vi "createILC.vi"() -> (3 "ILC":refnum<class "ILC.lvclass">)   [LabVIEW 2016]
uses:
  Common_ILC/ILC/ILC.lvclass
  Common_SerialProtocols/SerialCommunicator/SerialCommunicator.lvclass
  Common_SerialProtocols/SerialProtocolFactory/SerialProtocolFactory/SerialProtocolFactory.lvclass
  D:/Code/ts_dcabt/Common_SerialProtocols/SerialProtocolFactory/ISerialProtocolFactory/ISerialProtocolFactory.lvclass
  Model/ILCTC/ILCTC.lvclass
  D:/Code/ts_dcabt/Common_ILC/ILC/ILC.lvclass
  Common_SerialProtocols/SerialCommunicator/SerialCommunicator.lvclass/SerialCommunicator.ctl
  Common_ILC/ILC/ILC.lvclass/ILC.ctl
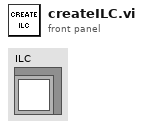
[diagram p1: front panel]
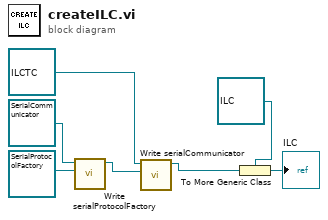
[diagram p0: block diagram]
diagram:
  n1 = call "Write serialProtocolFactory.vi"("serialProtocolFactory"=refnum<class "SerialProtocolFactory.lvclass"> refnum ("SerialProtocols.lvlib:SerialProtocolFactory.lvclass"), "SerialCommunicator in"=refnum<class "SerialCommunicator.lvclass"> refnum ("SerialProtocols.lvlib:SerialCommunicator.lvclass")) -> ("SerialCommunicator out"=w6:refnum<class "SerialCommunicator.lvclass">)  [unwired: 9 in]
  n2 = call "Write serialCommunicator.vi"("serialCommunicator"=w6, "ILC in"=refnum<class "ILCTC.lvclass"> refnum ("ILCTC.lvclass")) -> ("ILC out"=w2:refnum<class "ILCTC.lvclass">)  [unwired: 9 in]
  n3 = To More Generic Class(target class=refnum<class "ILC.lvclass"> refnum ("ILCCommon.lvlib:ILC.lvclass"), reference=w2) -> (generic class reference=→"ILC":refnum<class "ILC.lvclass">)
